vi "AxisUI2.vi"(10 "CardNumber":i32, 11 "IO Card Type":T1) -> ()   [LabVIEW 2019]
uses:
  IO Folder/IO_VI/IOCtrl/Ctrl/IO Card_Type.ctl
  Ctrl/right2.ctl
  Ctrl/left2.ctl
  Ctrl/down2.ctl
  Ctrl/Up2.ctl
  Ctrl/Teach2.ctl
  Ctrl/Move.ctl
  Ctrl/EmgStop.ctl
  Ctrl/SearchHome.ctl
  <vilib>/Utility/miscctls.llb/LVPointTypeDef.ctl
  LLB/Message/Ctrl/MsgDataInput.ctl
  LLB/Message/Ctrl/MsgPageSelect.ctl
  LLB/Message/Ctrl/LogType.ctl
  IO Folder/IO_VI/IOCtrl/Ctrl/DMC1000B_1 SelectOutput.ctl
  Axis_Class/AxisCard.lvclass
  Axis_Class/DMC 1000B/DMC_1000B.lvclass
  C:/Users/VIC/Desktop/204J1/204J1/System/Function/Axis/Axis_Class/AxisCard.lvclass
  Axis_Class/SubVI/Axis Motion/Axis_Jump Point.vi
  Axis_Class/SubVI/Axis Motion/Axis_Go Point.vi
  Axis_Class/SubVI/Axis Motion/Axis_Go Related.vi
  Axis_Class/SubVI/Axis Motion/Axis_Go Home.vi
  LLB/Commonly VI.lvlib
  LLB/Message/MsgShowAndLog.lvlib
  LLB/DMC3600/LTDMC.lvlib
panel:
  out "Axis Q":refnum<queue>
  out "Axis Q Name":string
  in  "Tab Control":enum32{"Page 1", "Page 2"}(tab)
  in  "Save Button":bool
  out "Actioning":bool
  in  "Btn_EmgStop":T2
  in  "Tab Control 2":T3(tab)
  out "Home Finish":T4 caption="Home"
  in  "SearchHome":T5
  in  "Btn_Move":T6
  in  "PointSelect":u16(ring) caption="點位選擇/PointSelect" items=["P0 - LHM", "P1 - LS1", "P2 - LS2", "P3 - LS3", "P4 - LS4", "P5 - LS5", "P6 - LS6", "P7 - LS7", "P8 - LS8", "P9 - AHM", "P10 - AS1", "P11 - AS2", "P12 - AS3", "P13 - AS4", "P14 - AS5", "P15 - AS6", "P16 - AS7", "P17 - AS8", "P18 - PHM", "P19 - PK1", "P20 - PK2", "P21 - PK3", "P22 - PK4", "P23 - PK5", "P24 - PK6", "P25 - PK7", "P26 - PK8"]
  in  "Btn_Teach":T7
  in  "Move Action":enum16{"Jump", "Go"}(ring) caption="移動方式/Mode"
  in  "Jog Distance Select":enum32{"Long", "Middle", "Short"}(radio)=enum."Middle" caption="寸動間距選擇(mm)/Jog Distance Select(mm)"
  in  "Current Position":T8 caption="當前位置/Current Position" {"Y3" format="%#.3f"; "X3" format="%#.3f"; "Y2" format="%#.3f"; "X2" format="%#.3f"; "Y1" format="%#.3f"; "X1" format="%#.2f"}
  in  "JogDistance":T8={"X1"=10.0, "Y1"=10.0, "X2"=10.0, "Y2"=10.0, "X3"=10.0, "Y3"=10.0} caption="寸動距離/JogDistance" {"Y3" min=0.01 max=100.0 format="%#.3f"; "X3" min=0.01 max=100.0 format="%#.3f"; "Y2" min=0.01 max=100.0 format="%#.3f"; "X2" min=0.01 max=100.0 format="%#.3f"; "Y1" min=0.01 max=100.0 format="%#.3f"; "X1" min=0.01 max=100.0 format="%#.3f"}
  in  "Jog":cluster{"X+":T9, "X-":T10, "Y-":T11, "Y+":T12} caption="寸動/Jog"
  in  "Station":enum16{"LineScan", "AI", "NGPick"}(ring)
  in  "AxisSpeed Basic":T13(array[cluster])=[{"AxisName"="Axis_0", "Accel"=0.5, "Deaccel"=0.5, "Speed"=40000.0, "Sramp"=0.4}, {"AxisName"="Axis_1", "Accel"=0.5, "Deaccel"=0.5, "Speed"=40000.0, "Sramp"=0.4}, {"AxisName"="Axis_2", "Accel"=0.5, "Deaccel"=0.5, "Speed"=40000.0, "Sramp"=0.4}, {"AxisName"="Axis_3", "Accel"=0.5, "Deaccel"=0.5, "Speed"=40000.0, "Sramp"=0.4}]
  in  "Tab Control 3":enum32{"Line Scan", "AI", "NG Pick"}(tab)
  in  "RobotPoint":string[][](table)=[["LHM", "0", "0", "0", "0", "", ""], ["LS1", "10", "10", "0", "0", "", ""], ["LS2", "75", "10", "0", "0", "", ""], ["LS3", "10", "160", "0", "0", "", ""], ["LS4", "75", "160", "0", "0", "", ""], ["LS5", "95", "10", "0", "0", "", ""], ["LS6", "160", "10", "0", "0", "", ""], ["LS7", "95", "160", "0", "0", "", ""], ["LS8", "160", "160", "0", "0", "", ""], ["AHM", "0", "0", "0", "0", "", ""], ["AS1", "20", "15", "20", "15", "", ""], ["AS2", "95", "15", "95", "15", "", ""], ["AS3", "20", "165", "20", "165", "", ""], ["AS4", "95", "165", "95", "165", "", ""], ["AS5", "115", "15", "115", "15", "", ""], ["AS6", "180", "15", "180", "15", "", ""], ["AS7", "115", "165", "115", "165", "", ""], ["AS8", "180", "165", "180", "165", "", ""], ["PHM", "0", "0", "0", "0", "", ""], ["PK1", "0", "0", "0", "0", "24", "10"], ["PK2", "0", "0", "0", "0", "99", "10"], ["PK3", "0", "0", "0", "0", "24", "160"], ["PK4", "0", "0", "0", "0", "99", "160"], ["PK5", "0", "0", "0", "0", "184", "10"], ["PK6", "0", "0", "0", "0", "259", "10"], ["PK7", "0", "0", "0", "0", "184", "160"], ["PK8", "0", "0", "0", "0", "259", "160"]]
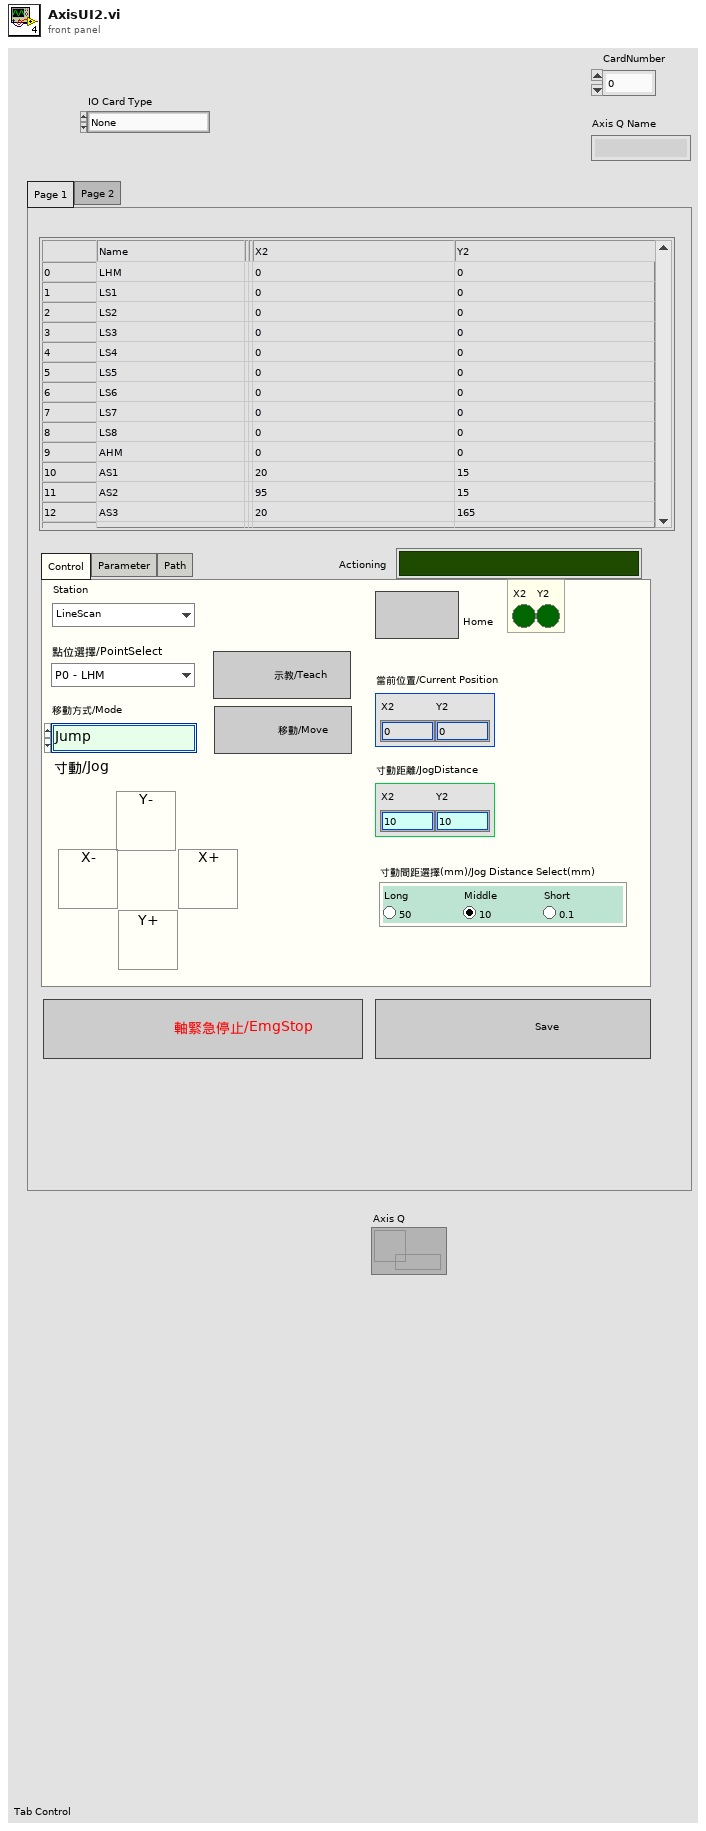
[diagram p1: front panel]
types:
  T1 = typedef "IO Card_Type.ctl" = enum16{"None", "Unidaq32", "6480", "2410C-64", "Zan", "DMC1000B", "16InOut", "Robot", "DMC3600"}
  T2 = typedef "EmgStop.ctl" = bool
  T3 = enum32{"Control", "PointEdit", "Parameter", "Path"}
  T4 = cluster{"Axis_0":bool, "Axis_1":bool, "Axis_2":bool, "Axis_3":bool, "Axis_2 2":bool, "Axis_3 2":bool}
  T5 = typedef "SearchHome.ctl" = bool
  T6 = typedef "Move.ctl" = bool
  T7 = typedef "Teach2.ctl" = bool
  T8 = cluster{"X1":dbl, "Y1":dbl, "X2":dbl, "Y2":dbl, "X3":dbl, "Y3":dbl}
  T9 = typedef "right2.ctl" = bool
  T10 = typedef "left2.ctl" = bool
  T11 = typedef "down2.ctl" = bool
  T12 = typedef "Up2.ctl" = bool
  T13 = cluster{"AxisName":string, "Accel":dbl, "Deaccel":dbl, "Speed":dbl, "Sramp":dbl}[]
  T14 = typedef "LVPointTypeDef.ctl" = cluster{"Horizontal":i16, "Vertical":i16}
  T15 = typedef "MsgDataInput.ctl" = cluster{"MsgPageSelect":T16, "LogType":T17, "Msg":string, "Time":string}
  T16 = typedef "MsgShowAndLog.lvlib/MsgPageSelect.ctl" = enum16{"System", "Comm", "IO", "Action", "Alarm"}
  T17 = typedef "MsgShowAndLog.lvlib/LogType.ctl" = enum16{"Auto", "Manual", "Handshake", "Error"}
  T18 = enum16{"Initial", "Load", "Save", "Read", "WriteSpeed", "WritePoint"}
  T19 = cluster{"Move Action":enum16{"Jump", "Go"}, "RingText.Text":string}
  T20 = cluster{"Move Action":enum16{"Jump", "Go"}, "trimmed string":string}
  T21 = cluster{"[0]":dbl, "[1]":dbl, "[2]":dbl, "[3]":dbl, "[4]":dbl, "[5]":dbl}
  T22 = cluster{"Home Finish[0]":bool, "Home Finish[1]":bool, "Home Finish[2]":bool, "Home Finish[3]":bool, "Home Finish[4]":bool, "Home Finish[5]":bool}
  T23 = cluster{"Current Position[0]":dbl, "Current Position[1]":dbl, "Current Position[2]":dbl, "Current Position[3]":dbl, "Current Position[4]":dbl, "Current Position[5]":dbl}
  T24 = typedef "DMC1000B_1 SelectOutput.ctl" = enum16{"M_Out0預備", "M_OUT01蜂鳴器", "M_OUT02紅燈", "M_OUT03綠燈", "M_OUT04黃燈", "M_OUT05上頂固定位氣缸電磁閥", "M_OUT06到料阻擋氣缸電磁閥", "M_OUT07向前機台發出要料#1信號", "M_OUT08向前機台發出要料#2信號", "M_OUT09向後機台發出有料#3信號", "M_OUT10向後機台發出有料#4信號", "M_OUT11接駁台馬達啟動開/關", "M_OUT12接駁台馬達慢速", "M_OUT13抽風機開/關", "M_OUT14上視覺上光源", "M_OUT15DC吹風扇開/關", "M_OUT16Z軸煞車釋放", "M_OUT17", "M_OUT18", "M_OUT19", "M_OUT20", "M_OUT21", "M_OUT22", "M_OUT23", "M_OUT24", "M_OUT25第一軸SEVON1伺服使能信號", "M_OUT26第二軸SEVON2伺服使能信號", "M_OUT27第三軸SEVON3伺服使能信號"}
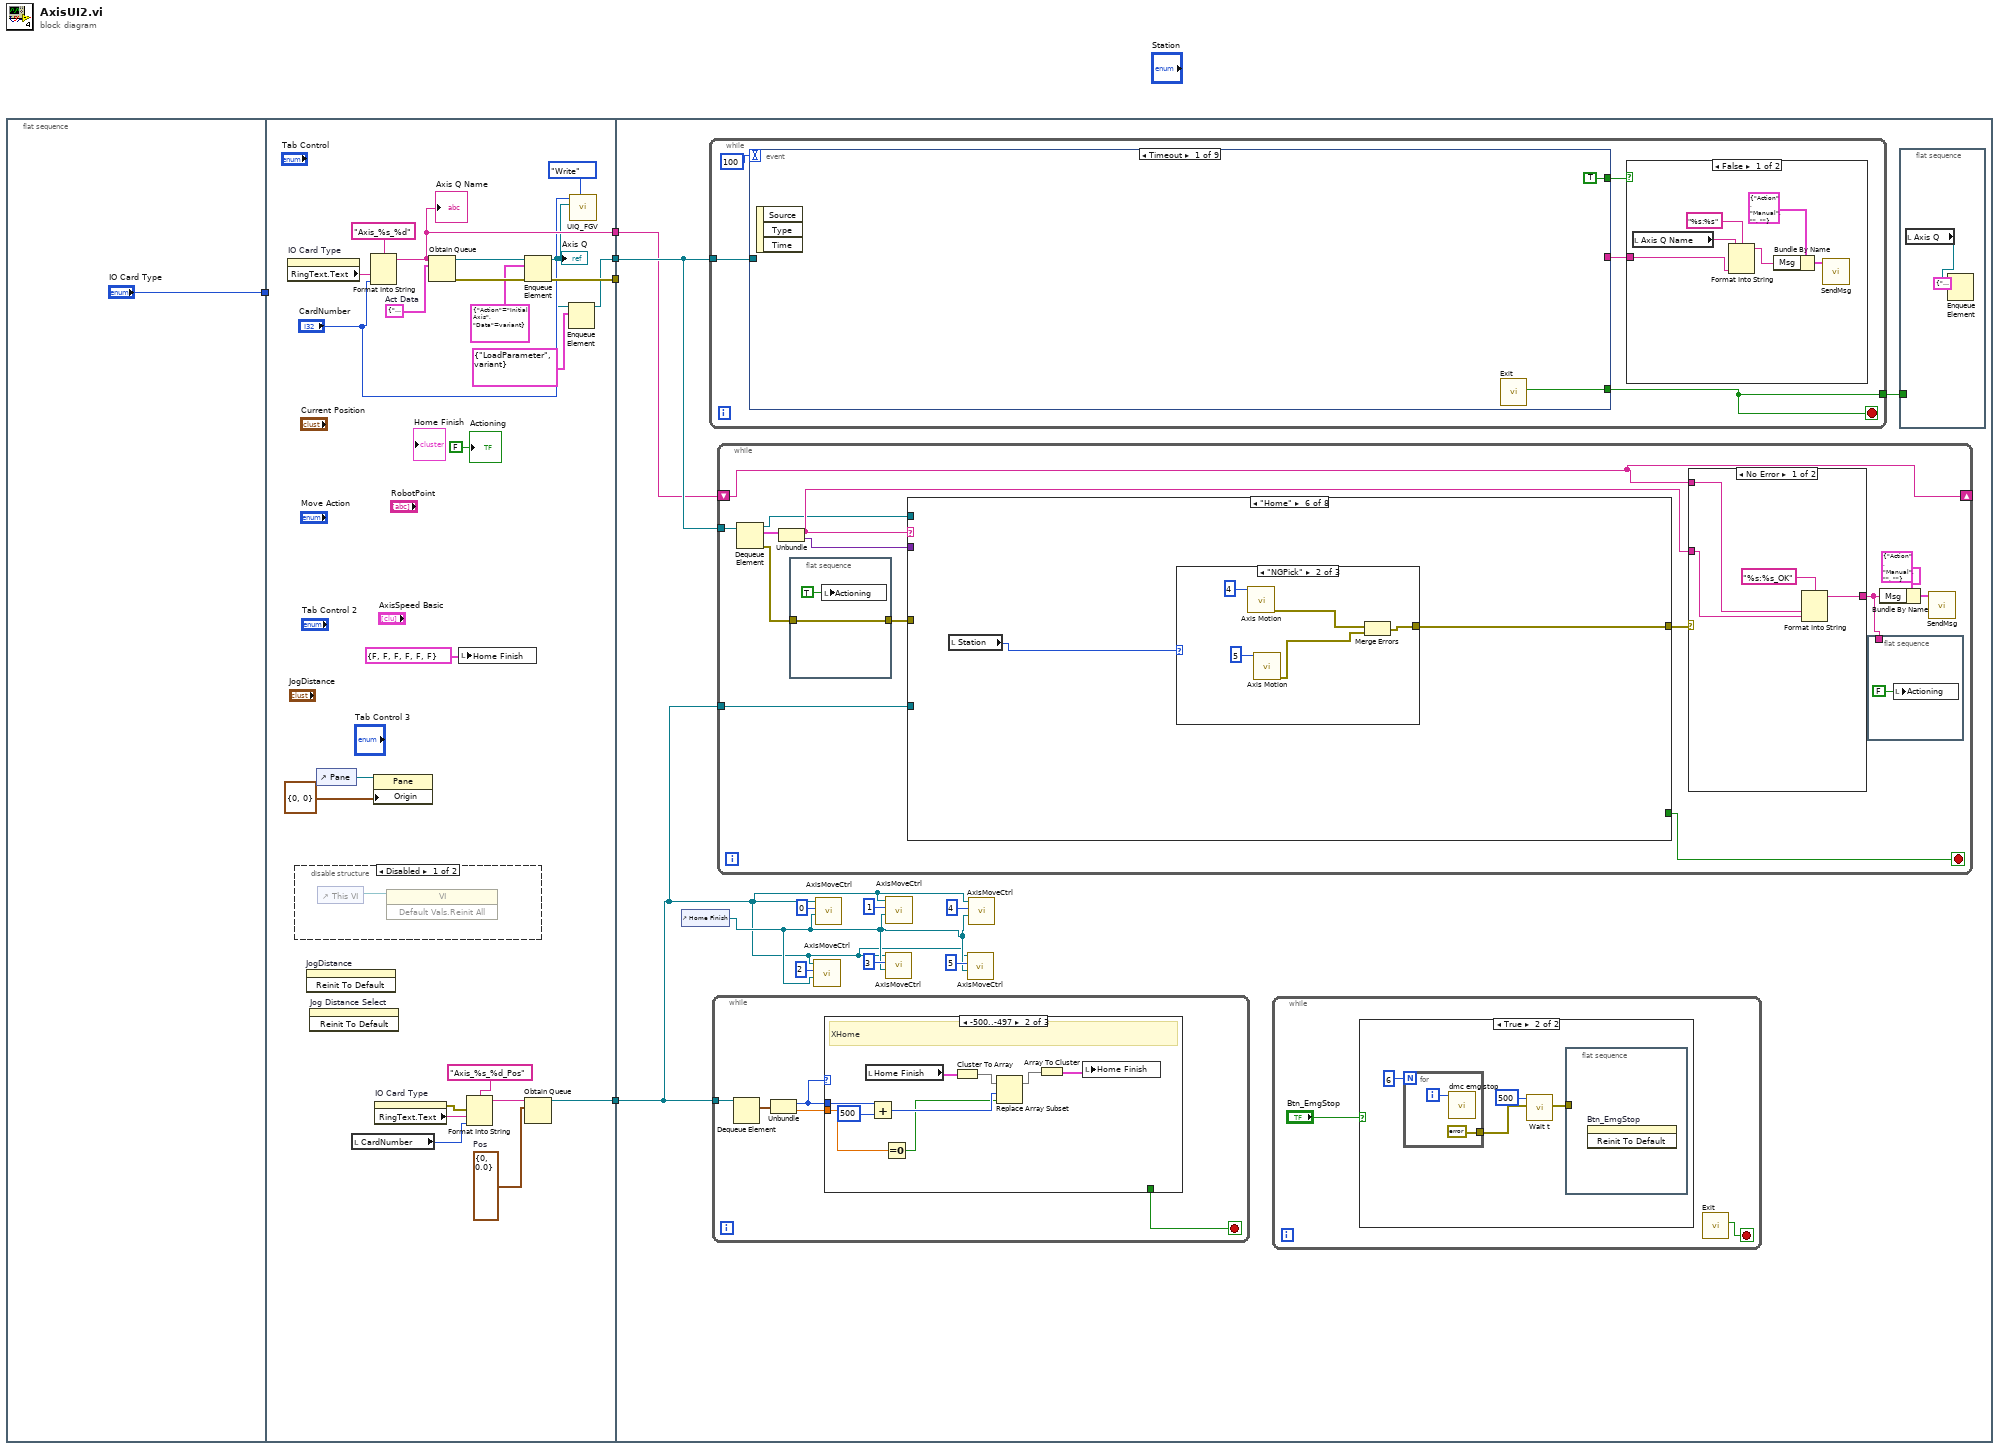
[diagram p0: block diagram]
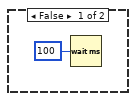
[diagram p3: hidden frame]
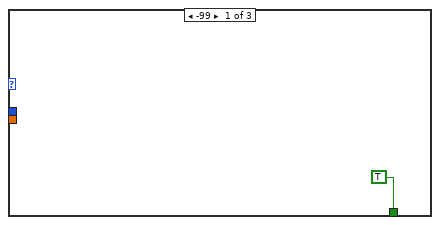
[diagram p4: hidden frame]
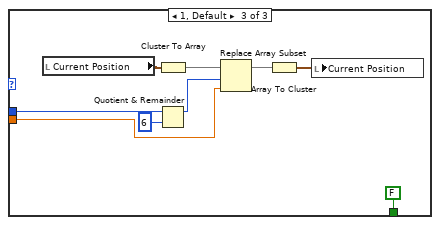
[diagram p5: hidden frame]
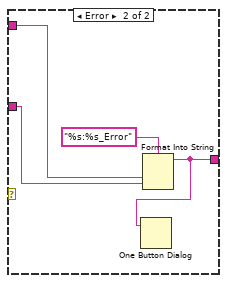
[diagram p6: hidden frame]
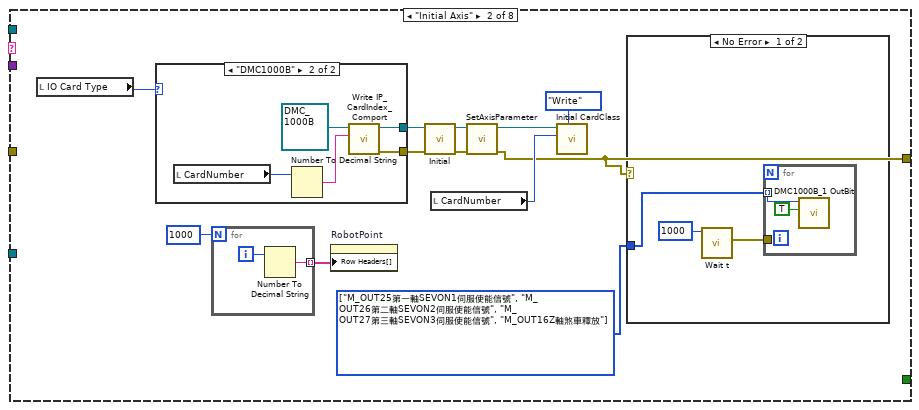
[diagram p8: hidden frame]
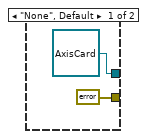
[diagram p10: hidden frame]
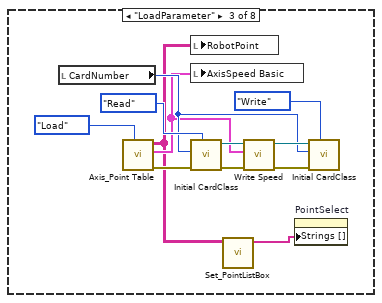
[diagram p11: hidden frame]
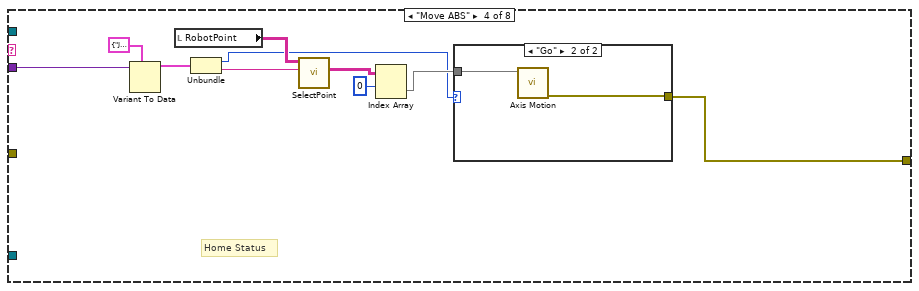
[diagram p12: hidden frame]
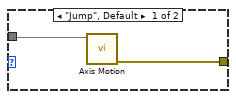
[diagram p13: hidden frame]
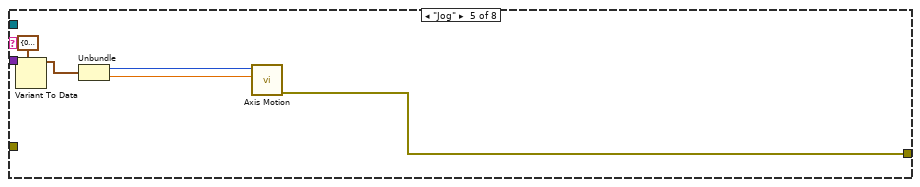
[diagram p14: hidden frame]
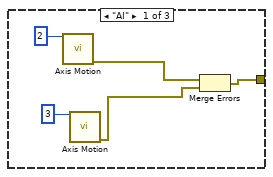
[diagram p15: hidden frame]
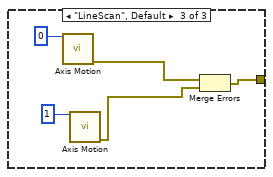
[diagram p16: hidden frame]
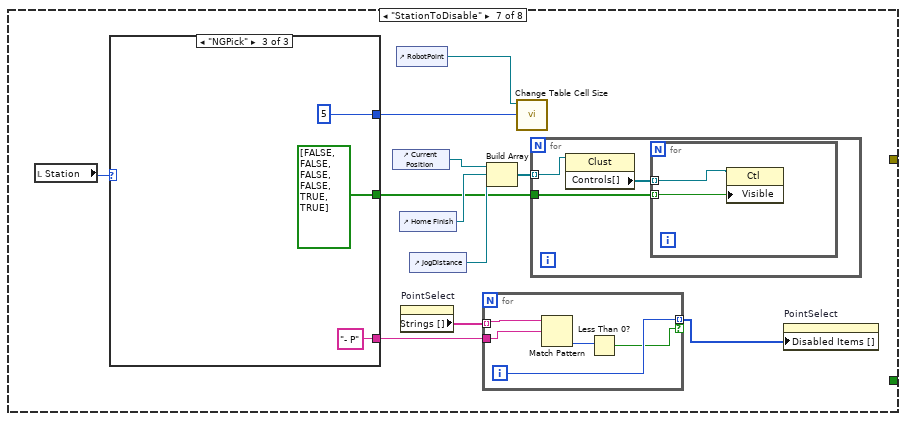
[diagram p17: hidden frame]
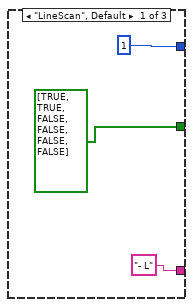
[diagram p18: hidden frame]
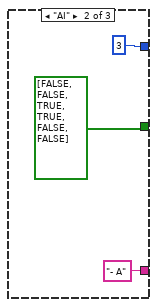
[diagram p19: hidden frame]
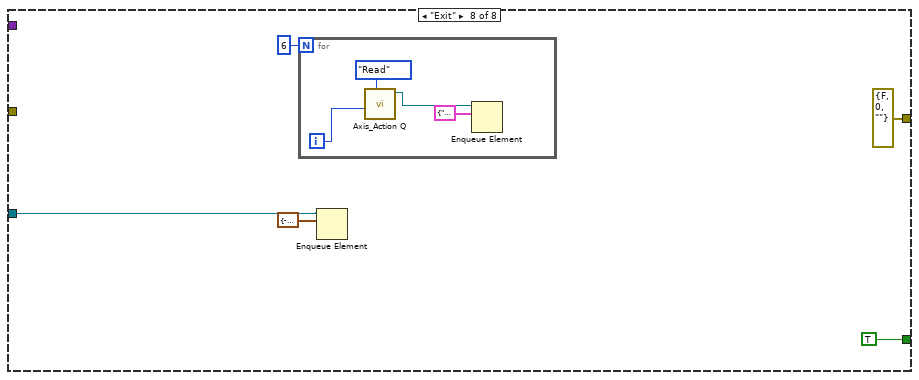
[diagram p20: hidden frame]
diagram:
  n1 = flat-sequence {
    tunnel: ["IO Card Type"] -> w1
    tunnel: [w9] -> w5
    tunnel: [w26] -> w4
    tunnel: [w19] -> w3
    tunnel: [w17] -> w2
    tunnel: w1 -> [_]
    tunnel: w5 -> [w41]
    tunnel: w4 -> [_]
    tunnel: w3 -> [w31]
    tunnel: w2 -> [w36]
    frame #0 {
    }
    frame #1 {
      w18 = cluster{"Action":string, "Data":variant} {"Action"="", "Data"=variant}  # Act Data
      w20 = cluster{"Axis":i32, "Pos":dbl} {"Axis"=0, "Pos"=0.0}  # Pos
      n2 = property on="IO Card Type" class="Enum (strict)"() -> ("RingText.Text"=w28:string)  [unwired: 2 in, 2 out]
      n3 = disable-structure shown="Disabled" {
        frame Disabled {
          n4 = control-ref of="This VI"() -> (w30:refnum<vi>)
          n5 = invoke class="VI" method="Default Vals.Reinit All"(reference=w30) -> ()  [unwired: 2 in, 3 out]
        }
        frame Enabled {
        }
      }
      n6 = invoke on="JogDistance" class="Clust (strict)" method="Reinit To Default"() -> ()  [unwired: 3 in, 3 out]
      n7 = invoke on="Jog Distance Select" class="RadioBtnsControl (strict)" method="Reinit To Default"() -> ()  [unwired: 3 in, 3 out]
      n8 = control-ref of="Pane"() -> (w15:refnum<vi>)
      n9 = local read "CardNumber"() -> (w21:i32)
      n10 = Format Into String(format string="Axis_%s_%d", w28, "CardNumber") -> (resulting string=w17:string)  [unwired: 2 in, 1 out]
      "Axis Q Name" <- w17
      n11 = property class="Pane"(reference=w15, "Origin"=T14 {"Horizontal"=0, "Vertical"=0}) -> ()  [unwired: 1 in, 2 out]
      n12 = property on="IO Card Type" class="Enum (strict)"() -> (error out=w23:errorcluster, "RingText.Text"=w22:string)  [unwired: 2 in, 1 out]
      n13 = Obtain Queue(name (unnamed)=w17, element data type=w18) -> (queue out=w27:refnum<queue>, error out=w26:errorcluster)  [unwired: 3 in, 1 out]
      n14 = local write "Home Finish"(T4 {"Axis_0"=FALSE, "Axis_1"=FALSE, "Axis_2"=FALSE, "Axis_3"=FALSE, "Axis_2 2"=FALSE, "Axis_3 2"=FALSE} ("Home Finish")) -> ()
      n15 = Format Into String(format string="Axis_%s_%d_Pos", error in=w23, w22, w21) -> (resulting string=w25:string)  [unwired: 1 in, 1 out]
      n16 = Enqueue Element(queue=w27, element=cluster{"Action":string, "Data":variant} {"Action"="Initial Axis", "Data"=variant}) -> (queue out=w8:refnum<queue>)  [unwired: 2 in, 2 out]
      "Axis Q" <- w8
      n17 = Obtain Queue(name (unnamed)=w25, element data type=w20) -> (queue out=w19:refnum<queue>)  [unwired: 3 in, 2 out]
      n18 = Enqueue Element(queue=w8, element=cluster{"Action":string, "Data":variant} {"Action"="LoadParameter", "Data"=variant}) -> (queue out=w9:refnum<queue>)  [unwired: 2 in, 2 out]
      n19 = call "UIQ_FGV.vi"("Enum"=enum16{"Initial", "Write", "Read"}."Write", "DataIn"=w8, "Index"="CardNumber") -> ()  [unwired: 8 in, 1 out]
      "Actioning" <- FALSE ("Actioning")
    }
    frame #2 {
      n20 = control-ref of="Home Finish"() -> (w32:refnum<vi>)
      n21 = while {
        tunnel: w41 -> [w217]
        tunnel: [w216] -> w35
        stop <- w216 stop-if-true
        n22 = event shown="[0] Timeout" {
          selector: _ -> [_ _ _ _ _ _ _ _ _]
          dyn-events: _ -> [_ _ _ _ _ _ _ _ _]
          timeout: 100 -> [_ _ _ _ _ _ _ _ _]
          tunnel: [w228 _ _ _ _ _ _ _ _] -> w216
          tunnel: [_ w233 w256 w270 _ "Axis Search Home" _ _ _] -> w219
          tunnel: [TRUE FALSE _ _ _ _ _ _ _] -> w218
          tunnel: w217 -> [_ _ w263 w279 _ w290 _ w304 _]
          event Timeout {
            n23 = event-data() -> ()  [unwired: 1 in, 3 out]
            n24 = call "Exit.vi"() -> ("ExitOut"=w228:bool)  [unwired: 11 in]
          }
          event Value Change {
            n25 = event-data() -> ()  [unwired: 1 in, 6 out]
            n26 = local read "Current Position"() -> (w250:T8)
            n27 = local read "PointSelect"() -> (w245:u16)
            n28 = property on="PointSelect" class="Ring (strict)"() -> ("Strings []"=w248:string[])  [unwired: 2 in, 2 out]
            n29 = Index Array(array=w248, index=w245) -> (element=w232:string)
            n30 = Cluster To Array(cluster=w250) -> (array=w249:dbl[])
            n31 = Match Pattern(string=w232, regular expression="-") -> (after substring=w231:string)  [unwired: 1 in, 3 out]
            n32 = Number To Fractional String(number=w249, precision (6)=i16 3) -> (F-format string=w235:string[])  [unwired: 2 in]
            n33 = property on="RobotPoint" class="Tbl (strict)"() -> ("Value"=w246:string[][])  [unwired: 2 in, 2 out]
            n34 = Build Array (concatenate)(w231, w235) -> (w247:string[])
            n35 = Index Array(array=w246, index (row)=w245) -> (element=w244:string[])  [unwired: 1 in]
            n36 = Replace Array Subset(array=w246, new element=w247, index (row)=w245) -> (w251:string[][])  [unwired: 1 in]
            n37 = property on="RobotPoint" class="Tbl (strict)"("Value"=w251) -> ()  [unwired: 2 in, 2 out]
            n38 = Array To Spreadsheet String(delimiter (Tab)=",", array=w244, 3:"%s" ("format string")) -> (spreadsheet string=w239:string)
            n39 = Array To Spreadsheet String(delimiter (Tab)=",", array=w235, 3:"%s" ("format string")) -> (spreadsheet string=w234:string)
            n40 = Concatenate Strings("Teach " ("string"), w239, "To " ("string"), w234) -> (w233:string)
          }
          event Value Change {
            w262 = cluster{"Action":string, "Data":variant} {"Action"="Move ABS", "Data"=variant}  # Act Data
            n41 = event-data() -> ()  [unwired: 1 in, 1 out]
            n42 = property on="PointSelect" class="Ring (strict)"() -> ("RingText.Text"=w258:string)  [unwired: 2 in, 2 out]
            n43 = local read "Move Action"() -> (w260:enum16{"Jump", "Go"})
            n44 = Match Pattern(string=w258, regular expression="-") -> (after substring=w254:string)  [unwired: 1 in, 3 out]
            n45 = call <vilib>:"Trim Whitespace.vi"("string"=w254) -> ("trimmed string"=w252:string)  [unwired: 1 in]
            n46 = Bundle("Move Action"=w260, "trimmed string"=w252) -> (w259:T20)  [unwired: 1 in]
            n47 = Bundle By Name(cluster=w262, "Data"=w259) -> (w261:cluster{"Action":string, "Data":variant})
            n48 = Enqueue Element(queue=w263, element=w261) -> ()  [unwired: 2 in, 3 out]
            n49 = property on="Move Action" class="Enum (strict)"() -> ("RingText.Text"=w253:string)  [unwired: 2 in, 2 out]
            n50 = Format Into String(format string="%s %s", w253, w252) -> (resulting string=w256:string)  [unwired: 2 in, 1 out]
          }
          event "Jog": Value Change {
            n51 = event-data() -> ("NewVal"=w278:cluster{"X+":T9, "X-":T10, "Y-":T11, "Y+":T12})  [unwired: 1 in, 1 out]
            n52 = local read "JogDistance"() -> (w276:T8)
            n53 = Cluster To Array(cluster=w278) -> (array=w277:T12[])
            n54 = Cluster To Array(cluster=w276) -> (array=w275:dbl[])
            n55 = call "Jog btn to Distance.vi"("Distance"=w275, "Jog Btn"=w277) -> ("Distance"=w269:dbl, "Axis"=w266:i32)  [unwired: 7 in, 1 out]
            n56 = local read "Station"() -> (w268:enum16{"LineScan", "AI", "NGPick"})
            n57 = Multiply(x=w268, y=2) -> (x*y=w267:i32)
            n58 = Add(x=w267, y=w266) -> (x+y=w265:i32)
            n59 = Bundle(w265, "Distance"=w269) -> (w272:cluster{i32, "Distance":dbl})  [unwired: 1 in]
            n60 = Bundle By Name(cluster=cluster{"Action":string, "Data":variant} {"Action"="Jog", "Data"=variant} ("element"), "Data"=w272) -> (w273:cluster{"Action":string, "Data":variant})
            n61 = Enqueue Element(queue=w279, element=w273) -> ()  [unwired: 2 in, 3 out]
            n62 = Format Into String(format string="Axis %d Jog %.3f", w265, w269) -> (resulting string=w270:string)  [unwired: 2 in, 1 out]
          }
          event "Jog Distance Select": Value Change {
            n63 = event-data() -> ()  [unwired: 1 in, 6 out]
            n64 = case shown="\"Short\"" "Jog Distance Select" {
              tunnel: [50.0 10.0 0.1] -> w283
              frame "Long", Default {
              }
              frame "Middle" {
              }
              frame "Short" {
              }
            }
            n65 = Initialize Array(w283, 6 ("dimension size")) -> (w281:dbl[])
            n66 = Array To Cluster(array=w281) -> (cluster=w280:T21)
            n67 = local write "JogDistance"(w280) -> ()
          }
          event Value Change {
            n68 = event-data() -> ()  [unwired: 1 in, 2 out]
            n69 = Enqueue Element(queue=w290, element=cluster{"Action":string, "Data":variant} {"Action"="Home", "Data"=variant}) -> ()  [unwired: 2 in, 3 out]
          }
          event "Save Button": Value Change {
            n70 = event-data() -> ()  [unwired: 1 in, 2 out]
            n71 = local read "RobotPoint"() -> (w291:string[][])
            n72 = local read "AxisSpeed Basic"() -> (w294:T13)
            n73 = call "Axis_Point Table.vi"("Enum"=T18."WritePoint", "PointIn"=w291) -> ("error Out"=w296:errorcluster)  [unwired: 7 in, 2 out]
            n74 = for {
              N: 6 -> [_]
              tunnel: w294 -> [w299] mode=indexing
              shift-right: [w300] -> w295
              shift-left: w296 -> [w301]
              i -> [w298]
              n75 = call "Axis_Point Table.vi"("Enum"=T18."WriteSpeed", "error In"=w301, "AxisData"=w299, "AxisIndex"=w298) -> ("error Out"=w300:errorcluster)  [unwired: 5 in, 2 out]
            }
            n76 = call "Axis_Point Table.vi"("Enum"=T18."Save", "error In"=w295) -> ()  [unwired: 7 in, 3 out]
          }
          event "Station": Value Change {
            n77 = event-data() -> ()  [unwired: 1 in, 1 out]
            n78 = Enqueue Element(queue=w304, element=cluster{"Action":string, "Data":variant} {"Action"="StationToDisable", "Data"=variant}) -> ()  [unwired: 2 in, 3 out]
          }
          event "PointSelect": Value Change {
            n79 = event-data() -> ("NewVal"=w307:u16)  [unwired: 1 in, 5 out]
            n80 = Bundle("NewVal"=w307, 0) -> (w306:cluster{"NewVal":u16, i32})  [unwired: 1 in]
            n81 = property on="RobotPoint" class="Tbl (strict)"("Index Values"=w306) -> ()  [unwired: 2 in, 2 out]
          }
        }
        n82 = case shown="False" w218 {
          tunnel: w219 -> [w222 _]
          frame False {
            n83 = local read "Axis Q Name"() -> (w224:string)
            n84 = Format Into String(format string="%s:%s", w224, w222) -> (resulting string=w221:string)  [unwired: 2 in, 1 out]
            n85 = Bundle By Name(cluster=T15 {"MsgPageSelect"=enum."Action", "LogType"=enum."Manual", "Msg"="", "Time"=""} ("DataIn"), "Msg"=w221) -> (w226:T15)
            n86 = call "SendMsg.vi"("DataIn"=w226) -> ()  [unwired: 10 in, 1 out]
          }
          frame True {
          }
        }
      }
      n87 = while {
        tunnel: w31 -> [w57]
        stop <- w53 stop-if-true
        n88 = Dequeue Element(queue=w57) -> (element=w56:cluster{"Axis":i32, "Pos":dbl})  [unwired: 2 in, 3 out]
        n89 = Unbundle(w56) -> ("Axis"=w54:i32, "Pos"=w55:dbl)
        n90 = case shown="-500..-497" w54 {
          tunnel: w54 -> [_ w65 w74]
          tunnel: w55 -> [_ w62 w71]
          tunnel: [TRUE _ FALSE] -> w53
          frame -99 {
          }
          frame -500..-497 {
            # "XHome"
            n91 = local read "Home Finish"() -> (w67:T4)
            n92 = Add(x=w65, y=500) -> (x+y=w63:i32)
            n93 = Equal To 0?(x=w62) -> (x = 0?=w61:bool)
            n94 = Cluster To Array(cluster=w67) -> (array=w66:bool[])
            n95 = Replace Array Subset(array=w66, new element=w61, index=w63) -> (w60:bool[])
            n96 = Array To Cluster(array=w60) -> (cluster=w59:T22)
            n97 = local write "Home Finish"(w59) -> ()
          }
          frame 1, Default {
            n98 = local read "Current Position"() -> (w76:T8)
            n99 = Cluster To Array(cluster=w76) -> (array=w75:dbl[])
            n100 = Quotient & Remainder(x=w74, y=6) -> (x-y*floor(x/y)=w72:i32)  [unwired: 1 out]
            n101 = Replace Array Subset(array=w75, new element=w71, index=w72) -> (w70:dbl[])
            n102 = Array To Cluster(array=w70) -> (cluster=w69:T23)
            n103 = local write "Current Position"(w69) -> ()
          }
        }
      }
      n104 = while {
        tunnel: w41 -> [w90]
        shift-right: [w83] -> _
        shift-left: w36 -> [w83]
        tunnel: w31 -> [w81]
        stop <- w82 stop-if-true
        n105 = Dequeue Element(queue=w90) -> (queue out=w80:refnum<queue>, element=w88:cluster{"Action":string, "Data":variant}, error out=w78:errorcluster)  [unwired: 2 in, 1 out]
        n106 = Unbundle(w88) -> ("Action"=w84:string, "Data"=w87:variant)
        n107 = flat-sequence {
          tunnel: [w93] -> w79
          tunnel: w78 -> [w93]
          frame #0 {
            n108 = local write "Actioning"(TRUE ("Actioning")) -> ()
          }
        }
        n109 = case shown="\"Home\"" w84 {
          tunnel: [_ w103 _ w140 w154 w160 _ errorcluster {"status"=FALSE, "code"=0, "source"=""} ("error IO")] -> w89
          tunnel: w87 -> [_ _ _ w148 w158 _ _ _]
          tunnel: [_ _ _ _ _ _ _ TRUE] -> w82
          tunnel: w81 -> [_ _ _ _ _ _ _ w208]
          tunnel: w80 -> [_ _ _ _ _ _ _ _]
          tunnel: w79 -> [_ _ _ _ _ _ _ _]
          frame "False", Default {
          }
          frame "Initial Axis" {
            w102 = T24[] [enum."M_OUT25第一軸SEVON1伺服使能信號", enum."M_OUT26第二軸SEVON2伺服使能信號", enum."M_OUT27第三軸SEVON3伺服使能信號", enum."M_OUT16Z軸煞車釋放"] items=["M_Out0預備", "M_OUT01蜂鳴器", "M_OUT02紅燈", "M_OUT03綠燈", "M_OUT04黃燈", "M_OUT05上頂固定位氣缸電磁閥", "M_OUT06到料阻擋氣缸電磁閥", "M_OUT07向前機台發出要料#1信號", "M_OUT08向前機台發出要料#2信號", "M_OUT09向後機台發出有料#3信號", "M_OUT10向後機台發出有料#4信號", "M_OUT11接駁台馬達啟動開/關", "M_OUT12接駁台馬達慢速", "M_OUT13抽風機開/關", "M_OUT14上視覺上光源", "M_OUT15DC吹風扇開/關", "M_OUT16Z軸煞車釋放", "M_OUT17", "M_OUT18", "M_OUT19", "M_OUT20", "M_OUT21", "M_OUT22", "M_OUT23", "M_OUT24", "M_OUT25第一軸SEVON1伺服使能信號", "M_OUT26第二軸SEVON2伺服使能信號", "M_OUT27第三軸SEVON3伺服使能信號"]
            n110 = local read "IO Card Type"() -> (w113:T1)
            n111 = case shown="\"DMC1000B\"" w113 {
              tunnel: [refnum<class "AxisCard.lvclass"> refnum ("AxisCard.lvclass") w124] -> w112
              tunnel: [errorcluster {"status"=FALSE, "code"=0, "source"=""} ("error out") w123] -> w111
              frame "None", Default {
              }
              frame "DMC1000B" {
                n112 = local read "CardNumber"() -> (w126:i32)
                n113 = Number To Decimal String(number=w126) -> (decimal integer string=w125:string)  [unwired: 1 in]
                n114 = call-dynamic "Write IP_CardIndex_Comport.vi"("IP/CardIndex/Comport"=w125, "AxisCard in"=refnum<class "DMC_1000B.lvclass"> refnum ("DMC_1000B.lvclass")) -> ("error out"=w123:errorcluster, "AxisCard out"=w124:refnum<class "DMC_1000B.lvclass">)  [unwired: 8 in]
              }
            }
            n115 = for {
              N: 1000 -> [_]
              tunnel: [w119] -> w104 mode=indexing
              i -> [w120]
              n116 = Number To Decimal String(number=w120) -> (decimal integer string=w119:string)  [unwired: 1 in]
            }
            n117 = property on="RobotPoint" class="Tbl (strict)"("Row Headers[]"=w104) -> ()  [unwired: 2 in, 2 out]
            n118 = call-dynamic "Initial.vi"("error in (no error)"=w111, "AxisCard in"=w112) -> ("error out"=w109:errorcluster, "AxisCard out"=w110:refnum<class "AxisCard.lvclass">)  [unwired: 8 in]
            n119 = local read "CardNumber"() -> (w106:i32)
            n120 = call-dynamic "SetAxisParameter.vi"("error in (no error)"=w109, "AxisCard in"=w110) -> ("error out"=w103:errorcluster, "AxisCard out"=w108:refnum<class "AxisCard.lvclass">)  [unwired: 8 in]
            n121 = call "Initial CardClass.vi"("Enum"=enum16{"Initial", "Write", "Read", "Exit"}."Write", "Card Number"=w106, "ClassIn"=w108) -> ()  [unwired: 7 in, 2 out]
            n122 = case shown="No Error" w103 {
              tunnel: w102 -> [w116 _]
              frame No Error {
                n123 = call "Wait t.vi"("wait(ms)"=u32 1000) -> ("error out"=w115:errorcluster)  [unwired: 10 in]
                n124 = for {
                  tunnel: w116 -> [w117] mode=indexing
                  tunnel: w115 -> [_]
                  n125 = call "DMC1000B_1 OutBit.vi"("BL"=TRUE, "IO_Output_1 Select"=w117) -> ()  [unwired: 9 in, 1 out]
                }
              }
              frame Error {
              }
            }
          }
          frame "LoadParameter" {
            n126 = local read "CardNumber"() -> (w135:i32)
            n127 = call "Axis_Point Table.vi"("Enum"=T18."Load") -> ("error Out"=w130:errorcluster, "AxisSpeed Basic"=w133:T13, "RobotPoint"=w129:string[][])  [unwired: 8 in]
            n128 = local write "RobotPoint"(w129) -> ()
            n129 = local write "AxisSpeed Basic"(w133) -> ()
            n130 = call "Initial CardClass.vi"("Enum"=enum16{"Initial", "Write", "Read", "Exit"}."Read", "error in"=w130, "Card Number"=w135) -> ("error Out"=w132:errorcluster, "DataOut"=w138:refnum<class "AxisCard.lvclass">)  [unwired: 7 in]
            n131 = call "Set_PointListBox.vi"("Table"=w129) -> ("Point"=w128:string[])  [unwired: 10 in]
            n132 = call-dynamic "Write Speed.vi"("error in (no error)"=w132, "AxisSpeed"=w133, "AxisCard in"=w138) -> ("error out"=w131:errorcluster, "AxisCard out"=w137:refnum<class "AxisCard.lvclass">)  [unwired: 7 in]
            n133 = property on="PointSelect" class="Ring (strict)"("Strings []"=w128) -> ()  [unwired: 2 in, 2 out]
            n134 = call "Initial CardClass.vi"("Enum"=enum16{"Initial", "Write", "Read", "Exit"}."Write", "error in"=w131, "Card Number"=w135, "ClassIn"=w137) -> ()  [unwired: 6 in, 2 out]
          }
          frame "Move ABS" {
            # "Home Status"
            n135 = Variant To Data(type=T19 {"Move Action"=enum."Jump", "RingText.Text"=""} ("output cluster"), Variant=w148) -> (data=w147:T19)  [unwired: 1 in, 1 out]
            n136 = local read "RobotPoint"() -> (w146:string[][])
            n137 = Unbundle(w147) -> ("Move Action"=w141:enum16{"Jump", "Go"}, "RingText.Text"=w145:string)
            n138 = call "SelectPoint.vi"("PointName"=w145, "RobotPointsTableIn"=w146) -> ("RobotPointsOut"=w144:string[][])  [unwired: 7 in, 2 out]
            n139 = Index Array(array=w144, index (row)=0) -> (element=w142:string[])  [unwired: 1 in]
            n140 = case shown="\"Go\"" w141 {
              tunnel: w142 -> [w150 w153]
              tunnel: [w151 w152] -> w140
              frame "Jump", Default {
                n141 = call-poly "Axis Motion.vi"("RobotPoints in"=w150) -> ("error out"=w151:errorcluster)  [unwired: 10 in]
              }
              frame "Go" {
                n142 = call-poly "Axis Motion.vi"("RobotPoints in"=w153) -> ("error out"=w152:errorcluster)  [unwired: 10 in]
              }
            }
          }
          frame "Jog" {
            n143 = Variant To Data(type=cluster{"Axis":i32, "Distance":dbl} {"Axis"=0, "Distance"=0.0} ("output cluster"), Variant=w158) -> (data=w157:cluster{"Axis":i32, "Distance":dbl})  [unwired: 1 in, 1 out]
            n144 = Unbundle(w157) -> ("Axis"=w156:i32, "Distance"=w155:dbl)
            n145 = call-poly "Axis Motion.vi"("Distance"=w155, "Axis Index"=w156) -> ("error"=w154:errorcluster)  [unwired: 9 in]
          }
          frame "Home" {
            n146 = local read "Station"() -> (w161:enum16{"LineScan", "AI", "NGPick"})
            n147 = case shown="\"NGPick\"" w161 {
              tunnel: [w162 w167 w172] -> w160
              frame "AI" {
                n148 = call-poly "Axis Motion.vi"("Axis Index"=2) -> ("error"=w164:errorcluster)  [unwired: 10 in]
                n149 = call-poly "Axis Motion.vi"("Axis Index"=3) -> ("error"=w163:errorcluster)  [unwired: 10 in]
                n150 = Merge Errors(w164, w163) -> (w162:errorcluster)
              }
              frame "NGPick" {
                n151 = call-poly "Axis Motion.vi"("Axis Index"=4) -> ("error"=w169:errorcluster)  [unwired: 10 in]
                n152 = call-poly "Axis Motion.vi"("Axis Index"=5) -> ("error"=w168:errorcluster)  [unwired: 10 in]
                n153 = Merge Errors(w169, w168) -> (w167:errorcluster)
              }
              frame "LineScan", Default {
                n154 = call-poly "Axis Motion.vi"("Axis Index"=0) -> ("error"=w174:errorcluster)  [unwired: 10 in]
                n155 = call-poly "Axis Motion.vi"("Axis Index"=1) -> ("error"=w173:errorcluster)  [unwired: 10 in]
                n156 = Merge Errors(w174, w173) -> (w172:errorcluster)
              }
            }
          }
          frame "StationToDisable" {
            n157 = local read "Station"() -> (w180:enum16{"LineScan", "AI", "NGPick"})
            n158 = case shown="\"NGPick\"" w180 {
              tunnel: [u32 1 ("Column") u32 3 ("Column") u32 5 ("Column")] -> w182
              tunnel: [bool[] [TRUE, TRUE, FALSE, FALSE, FALSE, FALSE] bool[] [FALSE, FALSE, TRUE, TRUE, FALSE, FALSE] bool[] [FALSE, FALSE, FALSE, FALSE, TRUE, TRUE]] -> w183
              tunnel: ["- L" "- A" "- P"] -> w178
              frame "LineScan", Default {
              }
              frame "AI" {
              }
              frame "NGPick" {
              }
            }
            n159 = control-ref of="Current Position"() -> (w184:refnum<vi>)
            n160 = control-ref of="RobotPoint"() -> (w181:refnum<vi>)
            n161 = control-ref of="Home Finish"() -> (w185:refnum<vi>)
            n162 = property on="PointSelect" class="Ring (strict)"() -> ("Strings []"=w179:string[])  [unwired: 2 in, 2 out]
            n163 = control-ref of="JogDistance"() -> (w186:refnum<vi>)
            n164 = for {
              tunnel: w179 -> [w192] mode=indexing
              tunnel: w178 -> [w191]
              tunnel: [w189] -> w177 mode=indexing if=w188
              i -> [w189]
              n165 = Match Pattern(string=w192, regular expression=w191) -> (offset past match=w190:i32)  [unwired: 1 in, 3 out]
              n166 = Less Than 0?(x=w190) -> (x < 0?=w188:bool)
            }
            n167 = Build Array(w184, w185, w186) -> (w187:refnum<vi>[])
            n168 = call "Change Table Cell Size.vi"("Column"=w182, "RobotPoint"=w181) -> ()  [unwired: 10 in]
            n169 = for {
              tunnel: w183 -> [w195]
              tunnel: w187 -> [w194] mode=indexing
              n170 = property class="Clust"(reference=w194) -> ("Controls[]"=w193:refnum<vi>[])  [unwired: 1 in, 2 out]
              n171 = for {
                tunnel: w195 -> [w197] mode=indexing
                tunnel: w193 -> [w196] mode=indexing
                n172 = property class="Ctl"(reference=w196, "Visible"=w197) -> ()  [unwired: 1 in, 2 out]
              }
            }
            n173 = property on="PointSelect" class="Ring (strict)"("Disabled Items []"=w177) -> ()  [unwired: 2 in, 2 out]
          }
          frame "Exit" {
            n174 = for {
              N: 6 -> [_]
              i -> [w212]
              n175 = call "Axis_Action Q.vi"("Enum"=enum16{"Initial", "Write", "Read"}."Read", "Axis Index"=w212) -> ("Axis ActQ Out"=w214:refnum<queue>)  [unwired: 7 in, 2 out]
              n176 = Enqueue Element(queue=w214, element=cluster{"Action":string, "Data":variant} {"Action"="Exit", "Data"=variant}) -> ()  [unwired: 2 in, 3 out]
            }
            n177 = Enqueue Element(queue=w208, element=cluster{"Axis":i32, "Pos":dbl} {"Axis"=-99, "Pos"=0.0}) -> ()  [unwired: 2 in, 3 out]
          }
        }
        n178 = case shown="No Error" w89 {
          tunnel: w84 -> [w96 w100]
          tunnel: [w95 w98] -> w77
          tunnel: w83 -> [w94 w99]
          frame No Error {
            n179 = Format Into String(format string="%s:%s_OK", w94, w96) -> (resulting string=w95:string)  [unwired: 2 in, 1 out]
          }
          frame Error {
            n180 = Format Into String(format string="%s:%s_Error", w99, w100) -> (resulting string=w98:string)  [unwired: 2 in, 1 out]
            n181 = One Button Dialog(message=w98) -> ()  [unwired: 1 in, 1 out]
          }
        }
        n182 = flat-sequence {
          tunnel: w77 -> [_]
          frame #0 {
            n183 = local write "Actioning"(FALSE ("Actioning")) -> ()
          }
        }
        n184 = Bundle By Name(cluster=T15 {"MsgPageSelect"=enum."Action", "LogType"=enum."Manual", "Msg"="", "Time"=""} ("DataIn"), "Msg"=w77) -> (w86:T15)
        n185 = call "SendMsg.vi"("DataIn"=w86) -> ()  [unwired: 10 in, 1 out]
      }
      n186 = call "AxisMoveCtrl.vi"("Home Finish"=w32, "Axis"=2, "PosQ"=w31) -> ()  [unwired: 9 in]
      n187 = call "AxisMoveCtrl.vi"("Home Finish"=w32, "Axis"=0, "PosQ"=w31) -> ()  [unwired: 9 in]
      n188 = call "AxisMoveCtrl.vi"("Home Finish"=w32, "Axis"=3, "PosQ"=w31) -> ()  [unwired: 9 in]
      n189 = call "AxisMoveCtrl.vi"("Home Finish"=w32, "Axis"=1, "PosQ"=w31) -> ()  [unwired: 9 in]
      n190 = call "AxisMoveCtrl.vi"("Home Finish"=w32, "Axis"=5, "PosQ"=w31) -> ()  [unwired: 9 in]
      n191 = call "AxisMoveCtrl.vi"("Home Finish"=w32, "Axis"=4, "PosQ"=w31) -> ()  [unwired: 9 in]
      n192 = while {
        stop <- w44 stop-if-true
        n193 = case shown="True" "Btn_EmgStop" {
          frame False {
            n194 = Wait (ms)(milliseconds to wait=u32 100) -> ()  [unwired: 1 out]
          }
          frame True {
            n195 = for {
              N: 6 -> [_]
              tunnel: [errorcluster {"status"=FALSE, "code"=0, "source"=""} ("error constant")] -> w48
              i -> [w52]
              n196 = call "dmc emg stop.vi"("CardNo"=w52) -> ()  [unwired: 9 in, 2 out]
            }
            n197 = call "Wait t.vi"("error in"=w48, "wait(ms)"=u32 500) -> ("error out"=w47:errorcluster)  [unwired: 9 in]
            n198 = flat-sequence {
              tunnel: w47 -> [_]
              frame #0 {
                n199 = invoke on="Btn_EmgStop" class="Bool" method="Reinit To Default"() -> ()  [unwired: 3 in, 3 out]
              }
            }
          }
        }
        n200 = call "Exit.vi"() -> ("ExitOut"=w44:bool)  [unwired: 11 in]
      }
      n201 = flat-sequence {
        tunnel: w35 -> [_]
        frame #0 {
          n202 = local read "Axis Q"() -> (w43:refnum<queue>)
          n203 = Enqueue Element(queue=w43, element=cluster{"Action":string, "Data":variant} {"Action"="Exit", "Data"=variant}) -> ()  [unwired: 2 in, 3 out]
        }
      }
    }
  }
